vi "Replace Control in VI.vi"   [LabVIEW 2021, in "EDT VI Script.lvlib"]
uses:
  EDT VI Script.lvlib
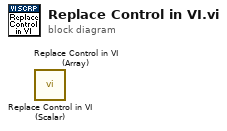
[diagram p0: block diagram]
diagram:
  n1 = call "Replace Control in VI (Scalar).vi"() -> ()  [unwired: 10 in, 2 out]
  n2 = call "Replace Control in VI (Array).vi"() -> ()  [unwired: 10 in, 2 out]
